vi "LogHeader.vi"() -> (3 "String":string)   [LabVIEW 2017, in "WaveformGenerator.lvlib"]
uses:
  WaveformGenerator.lvlib
  WaveformSpecs.ctl
panel:
  in  "Waveform Specification":T1
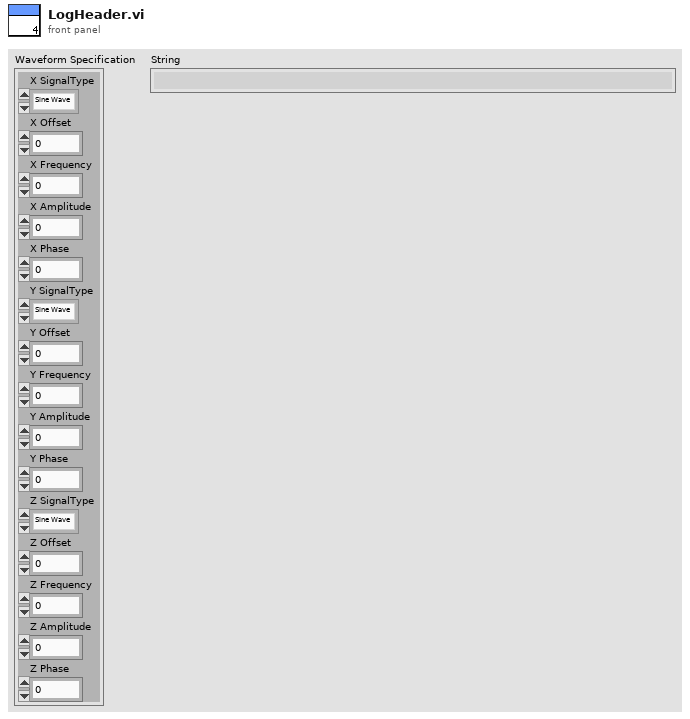
[diagram p1: front panel]
types:
  T1 = typedef "WaveformGenerator.lvlib/WaveformSpecs.ctl" = cluster{"X SignalType":enum16{"Sine Wave", "Triangle Wave", "Square Wave", "Sawtooth Wave"}, "X Offset":dbl, "X Frequency":dbl, "X Amplitude":dbl, "X Phase":dbl, "Y SignalType":enum16{"Sine Wave", "Triangle Wave", "Square Wave", "Sawtooth Wave"}, "Y Offset":dbl, "Y Frequency":dbl, "Y Amplitude":dbl, "Y Phase":dbl, "Z SignalType":enum16{"Sine Wave", "Triangle Wave", "Square Wave", "Sawtooth Wave"}, "Z Offset":dbl, "Z Frequency":dbl, "Z Amplitude":dbl, "Z Phase":dbl}
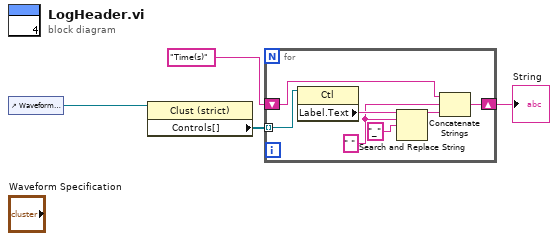
[diagram p0: block diagram]
diagram:
  n1 = control-ref of="Waveform Specification"() -> (w1:refnum<vi>)
  n2 = property class="Clust (strict)"(reference=w1) -> ("Controls[]"=w4:refnum<vi>[])  [unwired: 1 in, 2 out]
  n3 = for {
    tunnel: w4 -> [w11] mode=indexing
    shift-right: [w9] -> w2
    shift-left: "Time(s)" -> [w10]
    w5 = " " ("search string")
    n4 = property class="Ctl"(reference=w11) -> ("Label.Text"=w8:string)  [unwired: 1 in, 2 out]
    n5 = Search and Replace String(input string=w8, search string=w5, replace string="_" ("replace string (\"\")")) -> (result string=w6:string)  [unwired: 5 in, 3 out]
    n6 = Concatenate Strings(w10, w5, w6) -> (w9:string)
  }
  "String" <- w2
